vi "format output buffer.vi"(11 "read buffer":string) -> ()   [LabVIEW 2009]
uses:
  Range control watts.ctl
  Range control dBm.ctl
panel:
  out "Range dBm":T1
  out "Range W":T2
  out "number":i32
  out "Averaging?":string
  out "Range Type":string
  out "Mode (Unit)":string
  out "Status":string
  out "Range Scale":string
  out "Power num":dbl
  out "substring 2":string
  out "substring":string
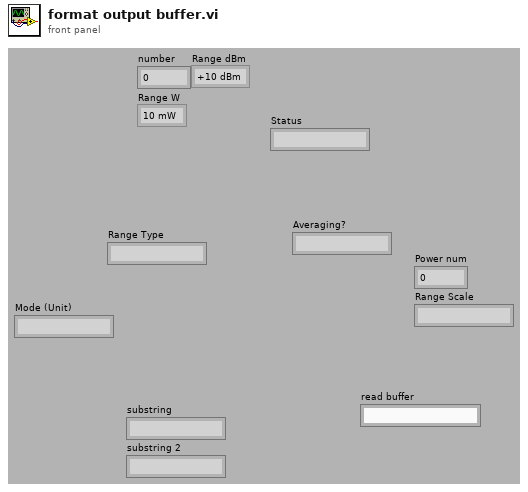
[diagram p1: front panel]
types:
  T1 = typedef "Range control dBm.ctl" = enum16{"+10 dBm", "0 dBm", "-10 dBm", "-20 dBm", "-30 dBm", "-40 dBm", "-50 dBm", "-60 dBm", "-70 dBm", "-80 dBm"}
  T2 = typedef "Range control watts.ctl" = enum16{"10 mW", "1 mW", "100 uW", "10 uW", "1 uW", "100 nW", "10 nW", "1 nW", "100 pW", "10 pW"}
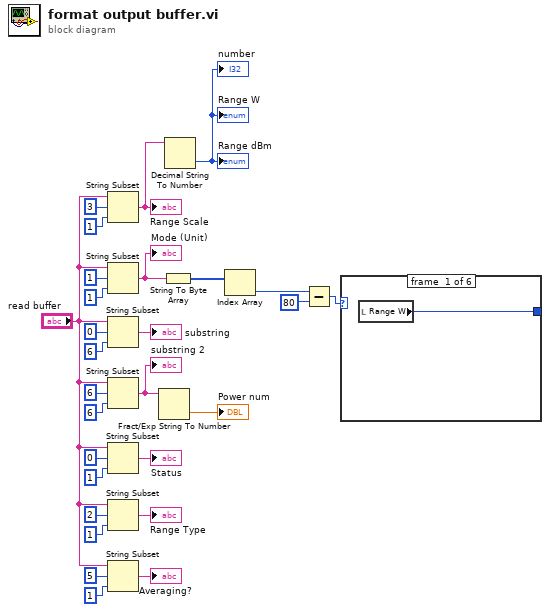
[diagram p0: block diagram]
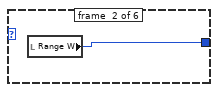
[diagram p2: hidden frame]
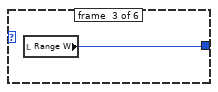
[diagram p3: hidden frame]
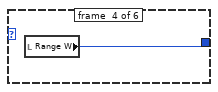
[diagram p4: hidden frame]
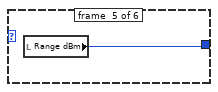
[diagram p5: hidden frame]
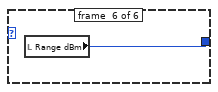
[diagram p6: hidden frame]
diagram:
  n1 = String Subset(string="read buffer", offset (0)=3, length (rest)=1 ("length (rest)")) -> (substring=w7:string)
  "Range Scale" <- w7
  n2 = String Subset(string="read buffer", offset (0)=1, length (rest)=1 ("length (rest)")) -> (substring=w6:string)
  "Mode (Unit)" <- w6
  n3 = String Subset(string="read buffer", offset (0)=0, length (rest)=6 ("length (rest)")) -> (substring=→"substring":string)
  n4 = String Subset(string="read buffer", offset (0)=6, length (rest)=6 ("length (rest)")) -> (substring=w23:string)
  "substring 2" <- w23
  n5 = String Subset(string="read buffer", offset (0)=0, length (rest)=1 ("length (rest)")) -> (substring=→"Status":string)
  n6 = String Subset(string="read buffer", offset (0)=2, length (rest)=1 ("length (rest)")) -> (substring=→"Range Type":string)
  n7 = String Subset(string="read buffer", offset (0)=5, length (rest)=1 ("length (rest)")) -> (substring=→"Averaging?":string)
  n8 = Fract/Exp String To Number(string=w23) -> (number=→"Power num":dbl)  [unwired: 3 in, 1 out]
  n9 = String To Byte Array(string=w6) -> (unsigned byte array=w5:u8[])
  n10 = Decimal String To Number(string=w7) -> (number=→"number" →"Range W" →"Range dBm":i32)  [unwired: 2 in, 1 out]
  n11 = Index Array(array=w5) -> (element=w4:u8)  [unwired: 1 in]
  n12 = Subtract(x=w4, y=u8 80) -> (x-y=w1:u8)
  n13 = case shown="5" w1 {
    tunnel: [w29 w30 w31 w32 w33 w34] -> _
    frame #0 {
      n14 = local read "Range W"() -> (w29:T2)
    }
    frame #1 {
      n15 = local read "Range W"() -> (w30:T2)
    }
    frame #2 {
      n16 = local read "Range W"() -> (w31:T2)
    }
    frame #3 {
      n17 = local read "Range W"() -> (w32:T2)
    }
    frame #4 {
      n18 = local read "Range dBm"() -> (w33:T1)
    }
    frame #5 {
      n19 = local read "Range dBm"() -> (w34:T1)
    }
  }
